vi "Configure Pulse Train.vi"(0 "VISA resource name":refnum<visa-resource-name>="USB0::0x05E6::0x2461::04090176::INSTR", 1 "Pulse Amplitude":dbl=1.0, 2 "Pulse Width":dbl=0.1, 3 "Pulse Off Time":dbl=0.1, 4 "Pulse Count":dbl=1.0, 5 "error in (no error)":errorcluster, 6 "Bias Level":dbl, 7 "Delay":dbl, 8 "Function (0:Voltage)":u16(ring) items=["Voltage", "Current"], 9 "Bias Limit":dbl=0.1, 10 "Buffer Name":string="defbuffer1", 11 "Pulse Limit":dbl=0.15, 12 "Fail Abort":bool=TRUE, 13 "Enable Measure":bool=TRUE) -> (14 "VISA resource name out":refnum<visa-resource-name>="USB0::0x05E6::0x2461::04090176::INSTR", 19 "error out":errorcluster)   [LabVIEW 2018, in "Keithley 2450.lvlib"]
doc: "This command defines a sequence of source pulses and to generate the pulse train.\n\n<B>This function is only compatible with the 2461.</B>"
uses:
  <instrlib>/Keithley 2450/Keithley 2450.lvlib
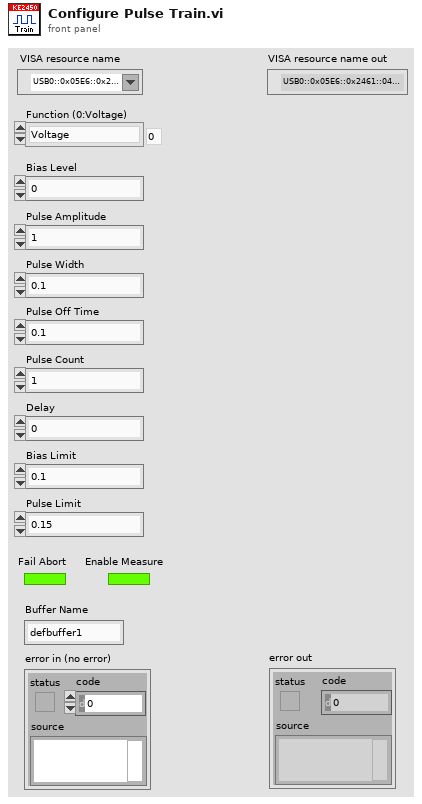
[diagram p1: front panel]
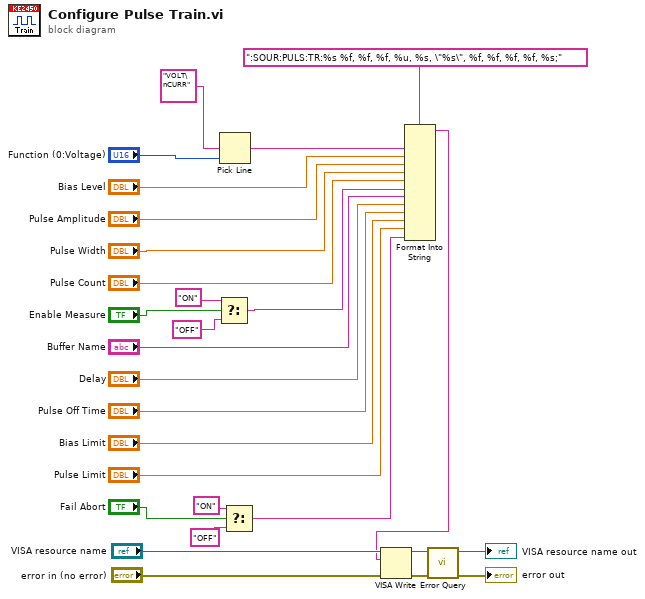
[diagram p0: block diagram]
diagram:
  n1 = Select(t="ON", s="Enable Measure", f="OFF") -> (s? t:f=w7:string)
  n2 = Pick Line(multi-line string="VOLT\nCURR", line index="Function (0:Voltage)") -> (output string=w18:string)  [unwired: 1 in]
  n3 = Select(t="ON", s="Fail Abort", f="OFF") -> (s? t:f=w1:string)
  n4 = Format Into String(format string=":SOUR:PULS:TR:%s %f, %f, %f, %u, %s, \"%s\", %f, %f, %f, %f, %s;" ("multi-line string"), w18, "Bias Level", "Pulse Amplitude", "Pulse Width", "Pulse Count", w7, "Buffer Name", "Delay", "Pulse Off Time", "Bias Limit", "Pulse Limit", w1) -> (resulting string=w20:string)  [unwired: 2 in, 1 out]
  n5 = VISA Write(VISA resource name="VISA resource name", write buffer=w20, error in (no error)="error in (no error)") -> (VISA resource name out=w24:refnum<visa-resource-name>, error out=w23:errorcluster)  [unwired: 1 out]
  n6 = call <instrlib>:"Error Query.vi"("error in (no error)"=w23, "VISA resource name"=w24) -> ("error out"=→"error out":errorcluster, "VISA resource name out"=→"VISA resource name out":refnum<visa-resource-name>)  [unwired: 8 out]
